vi "Machine_information.vi"() -> (1 "Machine:IP:Number":string[](array[string]), 2 "Machine:HD:Name":string[](array[string]))   [LabVIEW 2010]
uses:
  Globals/Constants_global.vi
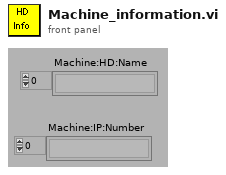
[diagram p1: front panel]
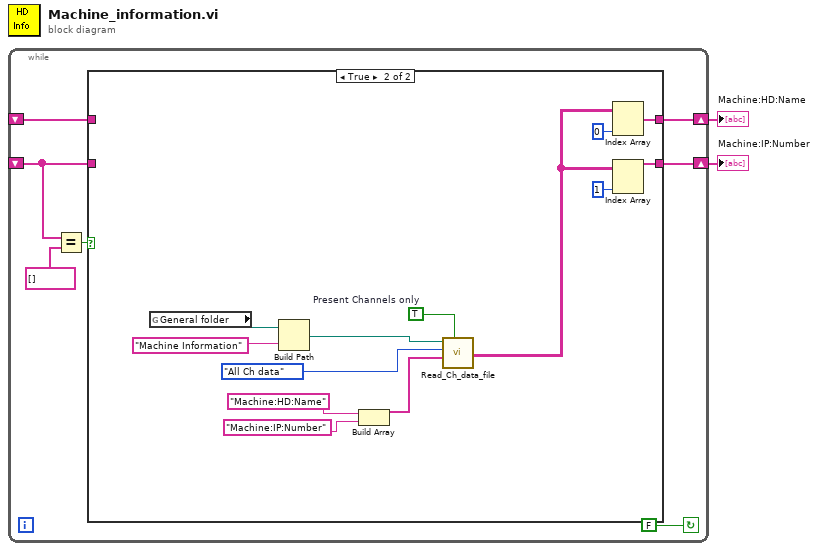
[diagram p0: block diagram]
diagram:
  n1 = while {
    shift-left: _ -> [w4]
    shift-right: [w9] -> w1
    shift-left: _ -> [w5]
    shift-right: [w8] -> w2
    stop <- FALSE continue-if-true
    n2 = Equal?(x=w4, y=string[] [] ("Channel Values")) -> (x = y?=w6:bool)
    n3 = case shown="True" w6 {
      tunnel: [w10 w18] -> w9
      tunnel: [w11 w17] -> w8
      tunnel: w5 -> [w11 _]
      tunnel: w4 -> [w10 _]
      frame False {
      }
      frame True {
        w16 = TRUE  # Present Channels only
        n4 = global read "Constants_global.vi" "General folder"() -> (w14:path)
        n5 = Build Path(base path=w14, name or relative path="Machine Information" ("Substring")) -> (appended path=w12:path)
        n6 = Build Array("Machine:HD:Name", "Machine:IP:Number") -> (w22:string[])
        n7 = call "Read_Ch_data_file.vi"("Present Channels only"=w16, "Present Channels"=w22, "Output"=enum16{"All Ch data", "The last few rows"}."All Ch data", "Filename"=w12) -> ("Channel Values"=w15:string[][])  [unwired: 1 in, 4 out]
        n8 = Index Array(array=w15, index (col)=0 ("Index")) -> (element=w17:string[])  [unwired: 1 in]
        n9 = Index Array(array=w15, index (col)=1 ("Index")) -> (element=w18:string[])  [unwired: 1 in]
      }
    }
  }
  "Machine:HD:Name" <- w2
  "Machine:IP:Number" <- w1
